vi "RSZVB Trace Data To Memory Trace.vi"(8 "error in (no error)":errorcluster {"code" format="%.0x"}, 9 "Data Trace (Trc1)":string="Trc1", 10 "Memory Trace (Mem1)":string="Mem1", 11 "VISA session":refnum<visa-resource-name>) -> (0 "error out":errorcluster {"code" format="%.0x"}, 3 "dup VISA session":refnum<visa-resource-name>)   [LabVIEW 2011]
doc: "This VI copies a data trace to a memory trace. The trace to be copied is specified as a trace with a name (string variable). The created memory trace is specified as a memory trace with an arbitrary name (string variable). An existing memory trace with the same name is overwritten.\n\nNote(s):\n\nThe copied trace is the data trace which is not modified by any mathematical operations. To copy a mathematical trace to a memory trace, use TRACe:COPY:MATH. To copy the active trace to the memory using an automatic memory trace name, use CALCulate<Ch/Tr>:MATH:MEMorize.\n\nRemote-control command(s):\nTRACe:COPY '<memory_trc>','<data_trc>'"
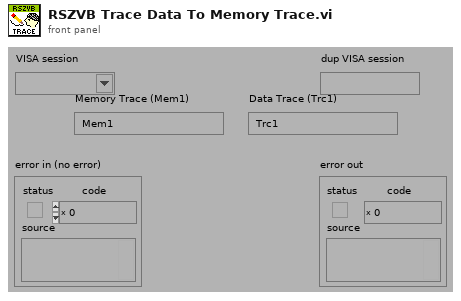
[diagram p1: front panel]
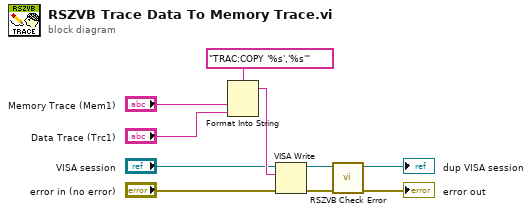
[diagram p0: block diagram]
diagram:
  n1 = Format Into String(format string="TRAC:COPY '%s','%s'", "Memory Trace (Mem1)", "Data Trace (Trc1)") -> (resulting string=w7:string)  [unwired: 2 in, 1 out]
  n2 = VISA Write(VISA resource name="VISA session", write buffer=w7, error in (no error)="error in (no error)") -> (VISA resource name out=w8:refnum<visa-resource-name>, error out=w9:errorcluster)  [unwired: 1 out]
  n3 = call "RSZVB Check Error.vi"("error in (no error)"=w9, "VISA session"=w8) -> ("error out"=→"error out":errorcluster, "dup VISA session"=→"dup VISA session":refnum<visa-resource-name>)  [unwired: 8 in]
